vi "Filter_Get all call chain parents.vi"(10 "Call Chain":string[](array[string]), 11 "Array":cluster{"Array":string[]}[](array[cluster])) -> (3 "parent indicies":i32[](array[numeric]))   [LabVIEW 2023]
doc: "For a given filtetr match, we need to take the call chain and break it down into all its parents and check fpor them. Spo for a call chain a,b,c, we check a,b,c; a,b; and a and retain those parent elements."
panel:
  out "Array 2":cluster{"Array":string[]}[](array[cluster])
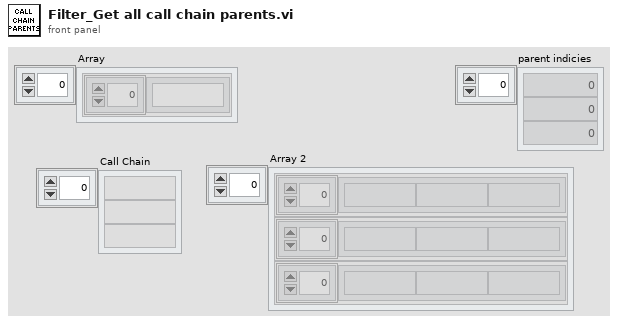
[diagram p1: front panel]
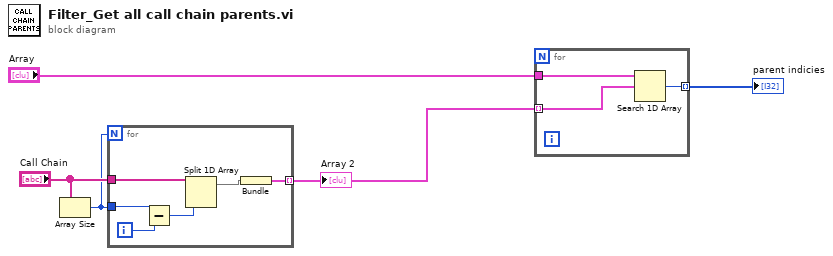
[diagram p0: block diagram]
diagram:
  n1 = Array Size(array="Call Chain") -> (size(s)=w2:i32)
  n2 = for {
    N: w2 -> [_]
    tunnel: "Call Chain" -> [w8]
    tunnel: w2 -> [w11]
    tunnel: [w6] -> w1 mode=indexing
    i -> [w10]
    n3 = Subtract(x=w11, y=w10) -> (x-y=w9:i32)
    n4 = Split 1D Array(array=w8, index=w9) -> (first subarray=w7:string[])  [unwired: 1 out]
    n5 = Bundle(w7) -> (w6:cluster{string[]})  [unwired: 1 in]
  }
  "Array 2" <- w1
  n6 = for {
    tunnel: [w14] -> w5 mode=indexing
    tunnel: "Array" -> [w13]
    tunnel: w1 -> [w12] mode=indexing
    n7 = Search 1D Array(1D array=w13, element=w12) -> (index of element=w14:i32)  [unwired: 1 in]
  }
  "parent indicies" <- w5
